vi "Dashboard Main.vi"() -> ()   [LabVIEW 2016]
uses:
  <vilib>/Rock Robotics/WPI/Camera/WPI_CameraSettings Read MJPG.ctl
  <vilib>/Rock Robotics/WPI/Camera/WPI_CameraImageSize.ctl
  HUD Time Slider.ctl
  <vilib>/Rock Robotics/WPI/DriverStation/WPI_DriverStationRobotMode2.ctl
  <vilib>/Rock Robotics/WPI/DriverStation/WPI_DriverStationAllianceInfo.ctl
  <vilib>/Rock Robotics/Network Tables/NT Read Numeric Array.vi
  <vilib>/Rock Robotics/Network Tables/NT Read Boolean.vi
  <vilib>/Rock Robotics/Network Tables/NT Write Numeric Array.vi
  <vilib>/event_ctls.llb/eventvkey.ctl
  <vilib>/Rock Robotics/WPI/Dashboard/WPI_DashboardLogging Global.vi
  <vilib>/Utility/miscctls.llb/LVRowAndColumnTypeDef.ctl
panel:
  out "CV LOCK":string
  out "Driver Control":bool
  out "Slide":T1 scale=0.0..100.0
  out "Robot Mode String":string
  out "Little Camera Image":T2(plugin-control)
  in  "TCP":refnum<k5>
  out "Robot IP":string
  out "Image Message":string="Timeout in Camera Communications"
  in  "Dashboard Tab":T3(tab)
  out "TALON ERR":bool
  out "VC ON":bool
  out "TEMP":dbl[unit](knob) scale=0.0..100.0
  out "AMPS":dbl(knob) caption="Gauge" scale=0.0..100.0
  out "Hopper Flaps":bool
  out "Hopper Down":bool
  out "Hopper Up":bool
  out "Intake Lock":bool
  out "Intake Active":bool
  out "Flaps":bool
  out "Gear Present":bool
  out "DeltaUS":dbl(knob) scale=-10.0..10.0
  out "ALIGN":bool caption="Boolean"
  out "Climb Motor Indicator":u32(colorbox)
  out "Intake Motor Indicator":u32(colorbox)
  out "Rear Right Indicator":u32(colorbox)
  out "Rear Left Indicator":u32(colorbox)
  out "Front Left Indicator":u32(colorbox)
  out "Front Right Indicator":u32(colorbox)
  out "BatPercentString":string
  out "BatteryPercent":u8(slide) scale=0.0..100.0
  out "BallSideActive":bool
  out "Mode":T4(ring)=enum."Auto Disabled"
  out "Gear is Front":bool
  out "Gear Auto Align":bool
  out "Auto Time Remaining":string
  out "INAV OK 2":bool
  out "CV OK":bool
  out "Auto Good":bool
  out "Robot Status":string
  out "Valid Autonomous Routines":i32(listbox)
  in  "AUTO SELECTION":i8(knob) scale=0.0..5.0
  out "Alliance Color":bool
  out "NT Connection":bool
  in  "Gear Side Camera Settings":T5={"fps"=30, "compression"=30, "Image Size"=enum."320x240", "Config Shown"=FALSE}
  in  "Ball Side Camera Settings":T5={"fps"=30, "compression"=30, "Image Size"=enum."320x240", "Config Shown"=FALSE}
  out "Ball Side Camera Info":cluster{bool, "Bandwidth (Mbps)":dbl, "FPS":dbl}
  out "Gear Side Camera Info":cluster{bool, "Bandwidth (Mbps)":dbl, "FPS":dbl}
  out "Big Camera Image":T2(plugin-control)
  # "HOPPER"
  # "A"
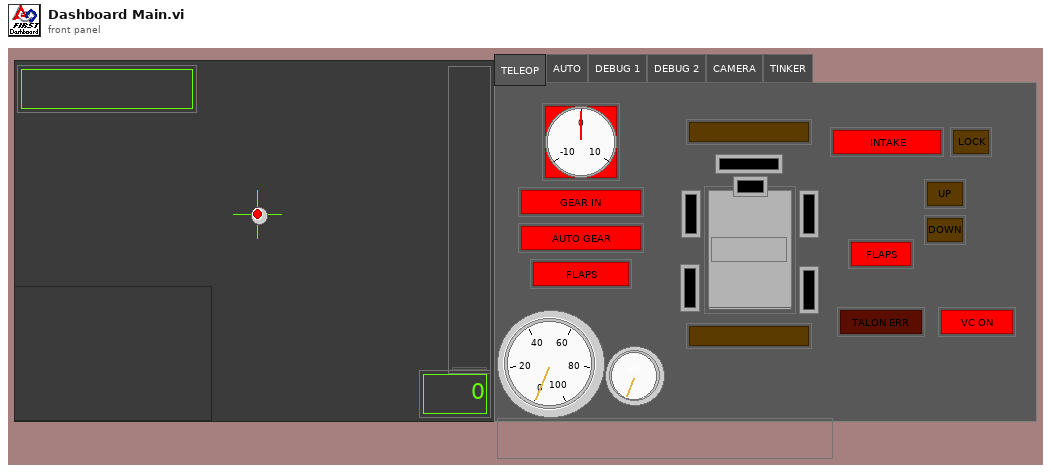
[diagram p1: front panel]
types:
  T1 = typedef "HUD Time Slider.ctl" = u8
  T2 = typedef "IMAQ Image.ctl" = refnum<image>
  T3 = enum32{"TELEOP", "AUTO", "DEBUG 1", "DEBUG 2", "CAMERA", "TINKER"}
  T4 = enum8{"Tele-Op Disabled", "Tele-Op Enabled", "Auto Disabled", "Auto Enabled", "Test Disabled", "Test Enabled", "Disconnected", "No Code", "E-Stop"}
  T5 = typedef "WPI_CameraSettings Read MJPG.ctl" = cluster{"fps":i32, "compression":i32, "Image Size":T6, "Config Shown":bool}
  T6 = typedef "WPI_CameraImageSize.ctl" = enum16{"640x480", "320x240", "160x120", "Custom"}
  T7 = typedef "Image Type" = u32
  T8 = cluster{"IDs":cluster{"RPC field ID":u16, "Unique ID":u16}, "String":string}
  T9 = enum32{"Drive", "Camera", "Basic", "Custom", "Test", "Commands", "Checklist", "Variables"}
  T10 = cluster{"Operation":enum16{"Update", "Clear"}, "Color Box":u32}[]
  T11 = typedef "eventvkey.ctl" = enum16{"ASCII", "Enter", "Return", "Shift", "Ctrl", "Alt", "Cmd", "Opt", "Caps", "NumLock", "Clear", "Break", "Up", "Down", "Left", "Right", "Insert", "Delete", "Home", "End", "PageUp", "PageDown", "Escape", "Help", "Pause", "ScrollLock", "F1", "F2", "F3", "F4", "F5", "F6", "F7", "F8", "F9", "F10", "F11", "F12", "F13", "F14", "F15", "F16", "F17", "F18", "F19", "F20", "F21", "F22", "F23", "F24", "Play", "VolumeUp", "VolumeDown", "Mute", "Two Byte Char"}
  T12 = cluster{"Image Size":bool, "Image Type":bool, "Pixel Value":bool, "ROI Information":bool, "Zoom Factor":bool}
  T13 = typedef "WPI_DriverStationRobotMode2.ctl" = enum16{"Autonomous Disabled", "Autonomous Enabled", "Teleop Disabled", "Teleop Enabled", "Disconnected", "Finish", "Test Disabled", "Test Enabled", "Emergency Stopped"}
  T14 = typedef "WPI_DriverStationAllianceInfo.ctl" = enum16{"Red", "Blue", "Invalid"}
  T15 = cluster{"Operation":enum16{"Update", "Clear"}, "Color Box":u32}
  T16 = typedef "LVRowAndColumnTypeDef.ctl" = cluster{"Row":i32, "Column":i32}
  T17 = cluster{"Test Progress":u8, "Test Progress Text":string}
  T18 = typedef "WPI_DriverStationPositionInfo.ctl" = enum16{"1", "2", "3"}
  T19 = cluster{"Error Strings":string, "Disable Counts":cluster{u16, u16}, "Rail Faults":cluster{u16, u16, u16}, "Robot IP":string, "DB Mode":u8, "Event Info":cluster{"Name":string, "Type":u8, "Number":u16, "Replay":u8}}
  T20 = cluster{"Storage":cluster{"Disk Free":u64, "RAM Block":u32, "RAM free":u32}, "CPU Utilization":cluster{"CPU % ISR":sgl, "CPU % Time Crit":sgl, "CPU % Timed Str":sgl, "CPU % High":sgl, "CPU % Above":sgl, "CPU % Normal":sgl, "CPU % Low":sgl}, "CAN":cluster{"% Bus Utilization":sgl, "Bus Off Cnt":u32, "TX_FIFO Full Cnt":u32, "Receive Error Cnt":u8, "Transmit Error Cnt":u8}, "HID":cluster{"HID Outputs":u32, "Rumble Low":u16, "Rumble High":u16}[]}
  T21 = cluster{"Status bits":cluster{"Test Mode":bool, "Autonomous":bool, "Enabled":bool, "Code Start":bool, "Brownout":bool, "Reserved 2":bool, "Reserved 3":bool, "E-Stop":bool}, "Code Trace":cluster{"Disabled":bool, "TeleOp":bool, "Auto":bool, "Test":bool}, "Controller Type":enum16{"unknown", "cRIO", "roboRio"}, "Code?":enum16{"unknown", "noCode", "code"}, "Battery V":dbl}
  T22 = cluster{"Control Bits":cluster{"TestMode":bool, "Autonomous":bool, "Enabled":bool, "FMS Present":bool, bool, bool, bool, "E-Stop":bool}, "Team Station ":u8, "Countdown":sgl, "Joystick Values":cluster{"Axes":dbl[], "Buttons":bool[], "POVs":i16[]}[]}
  T23 = cluster{"Axes":dbl[], "Buttons":bool[], "POVs":i16[]}[]
  T24 = cluster{"Axes":dbl[], "Buttons":bool[], "POVs":i16[]}
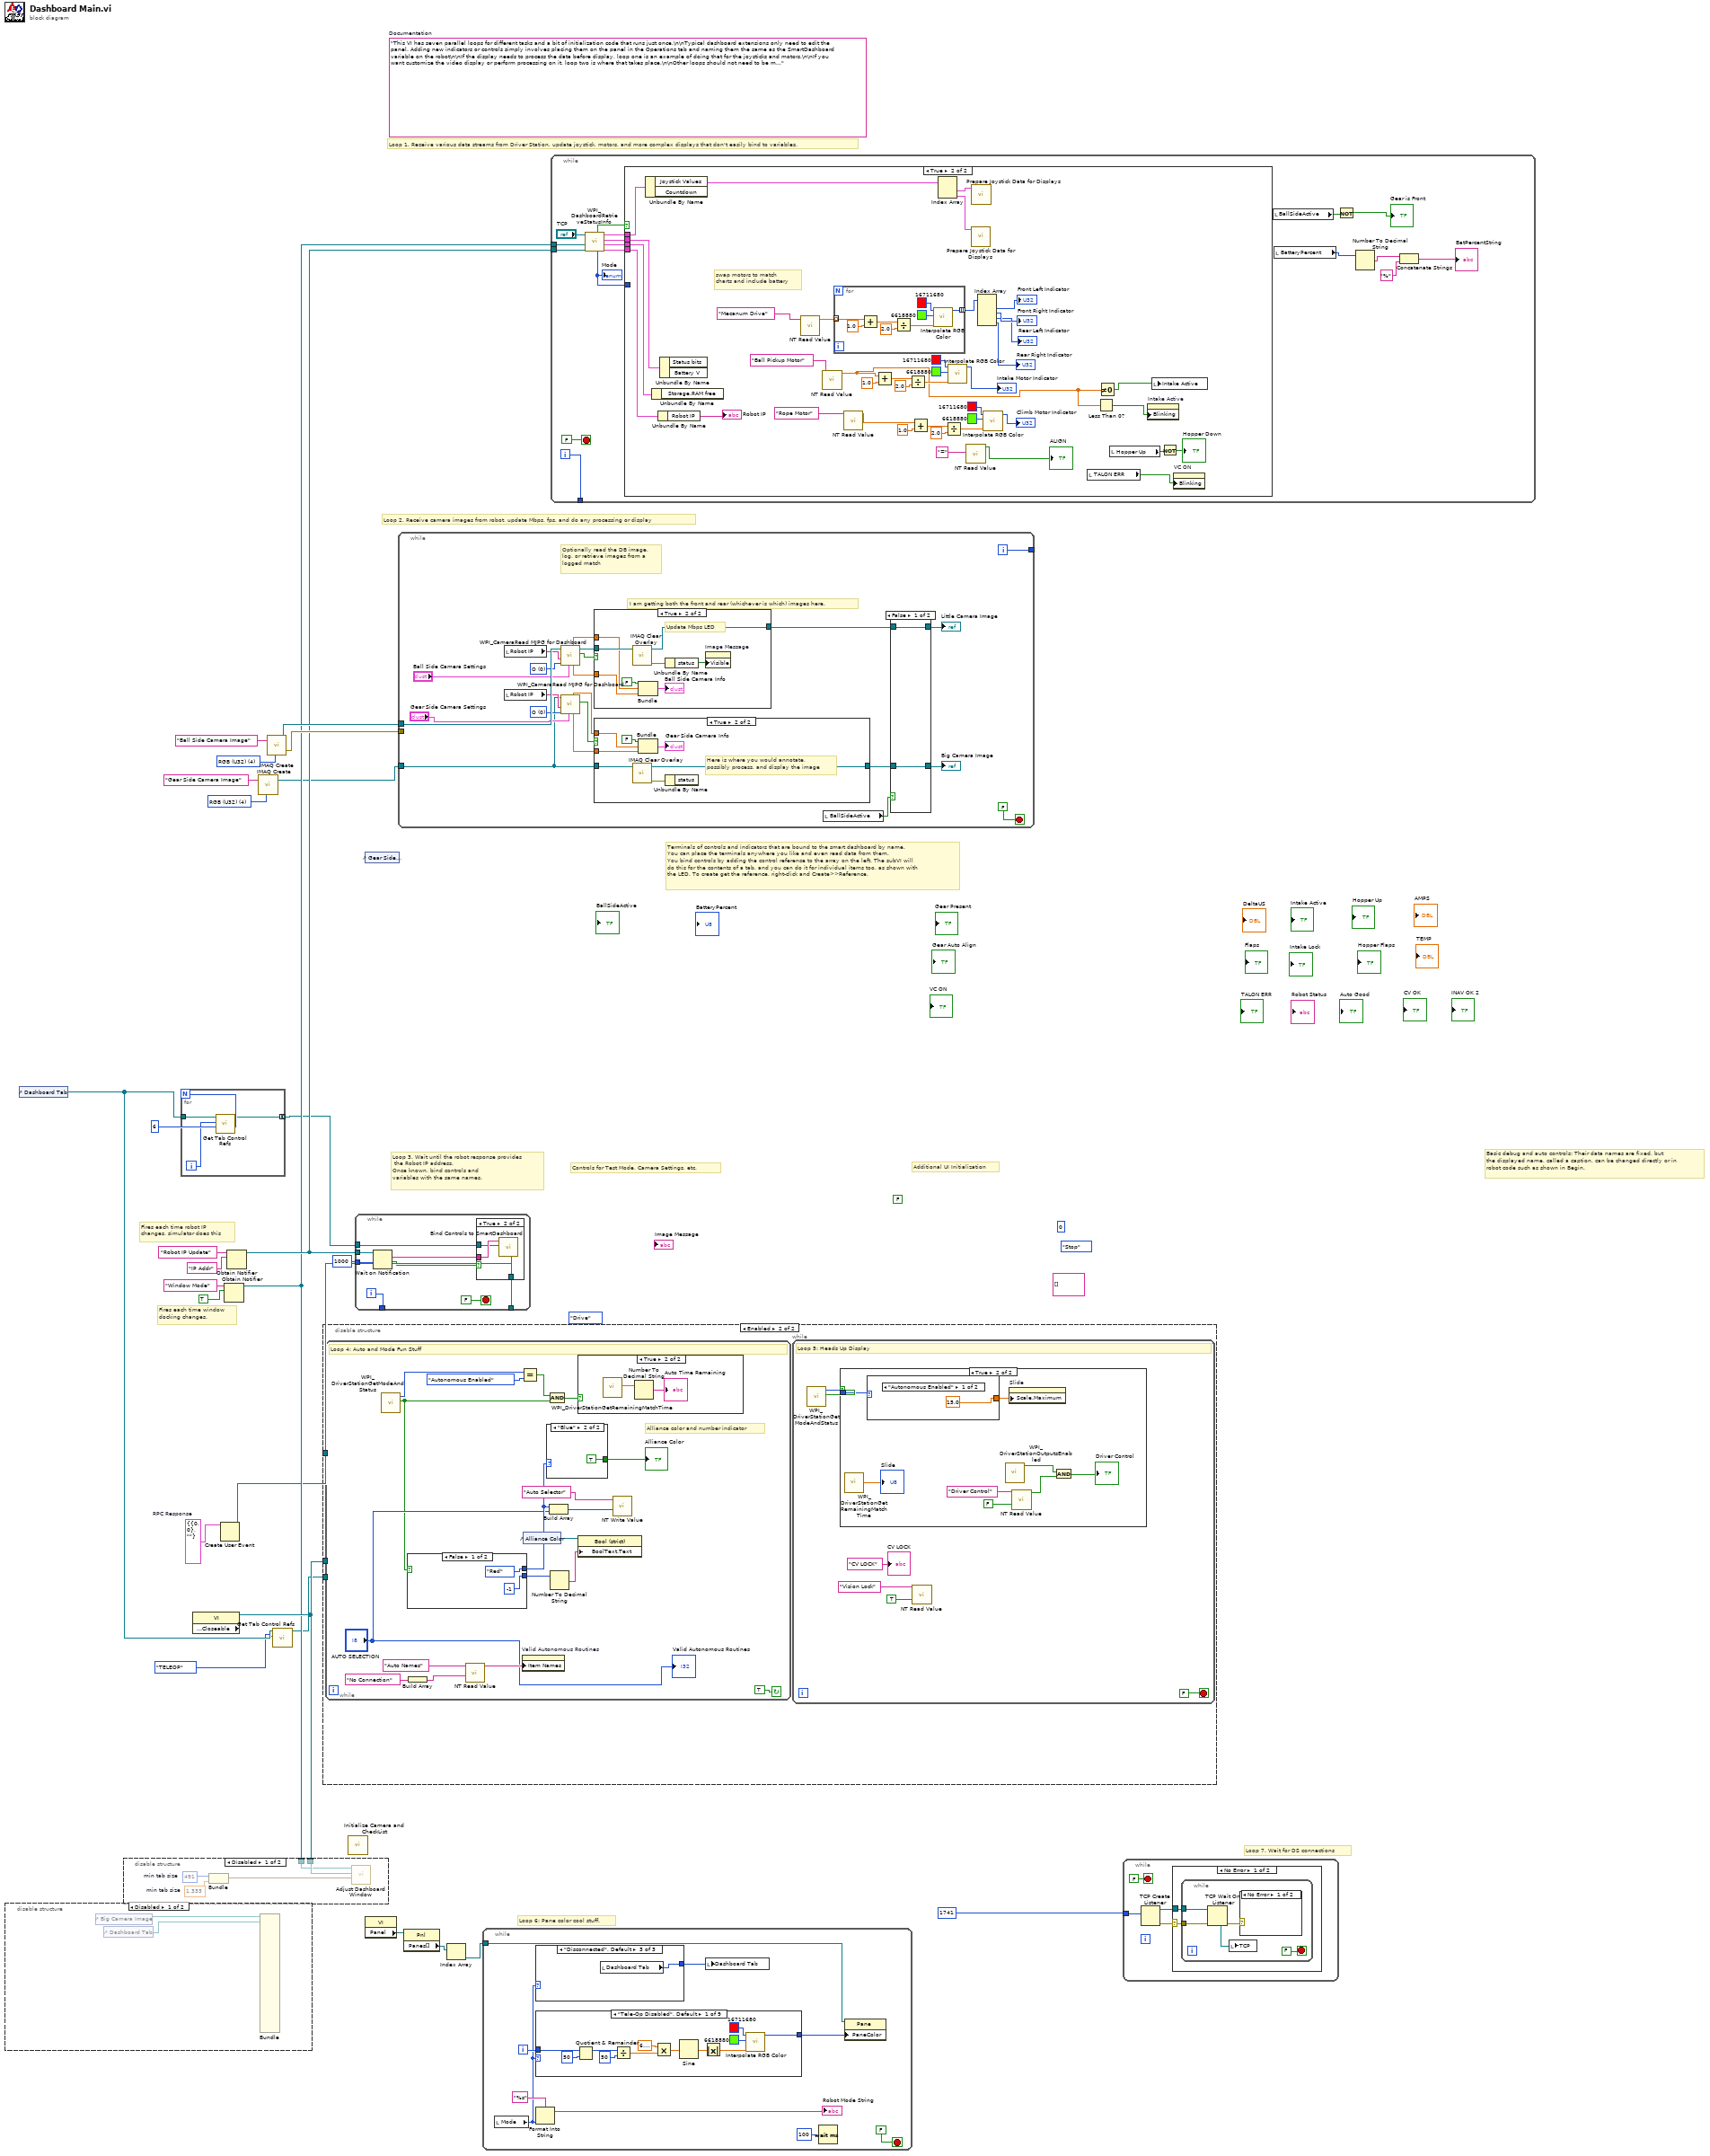
[diagram p0: block diagram]
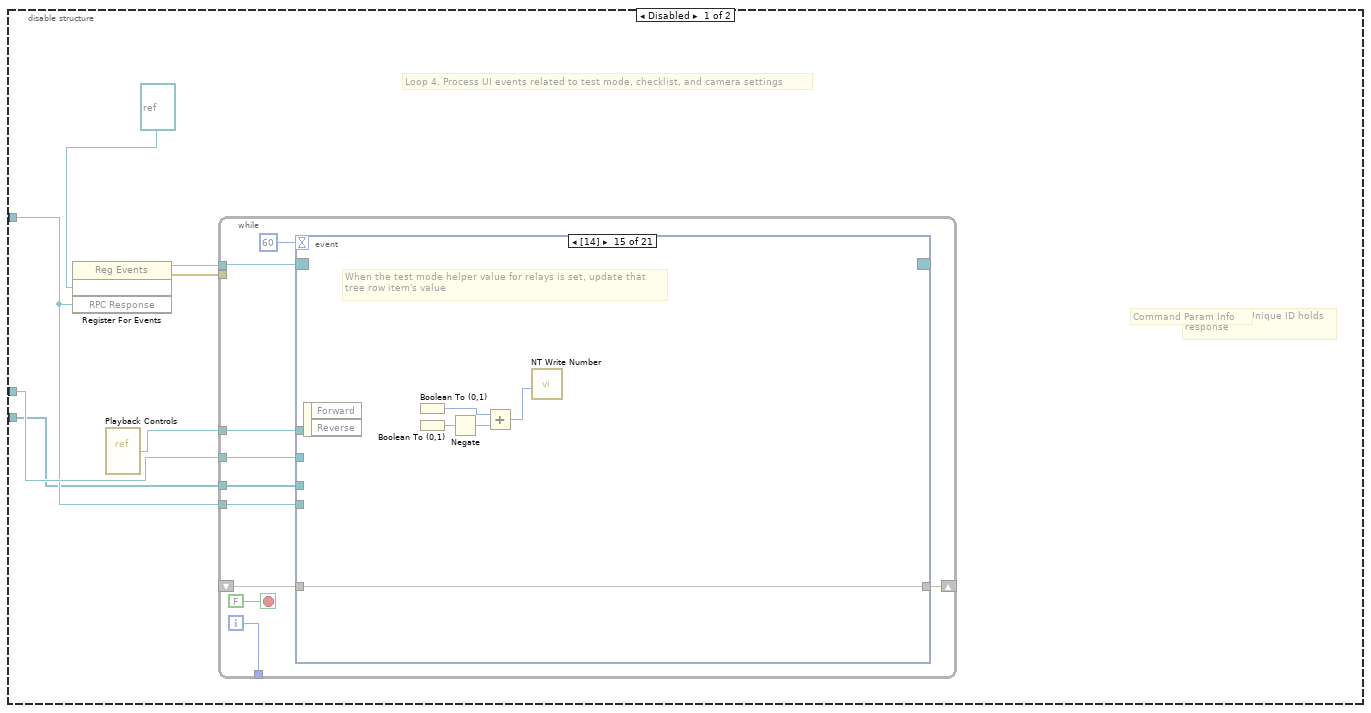
[diagram p4: hidden frame]
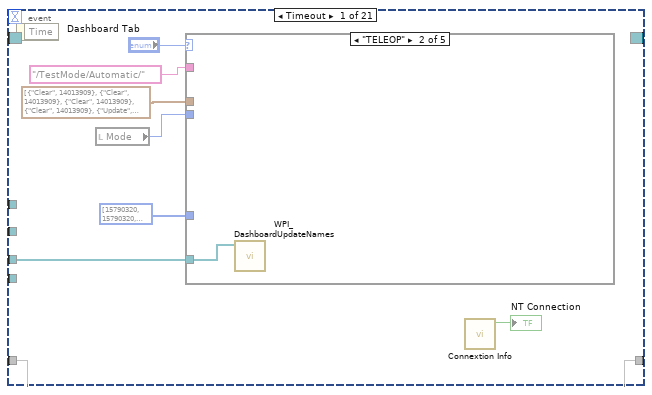
[diagram p5: hidden frame]
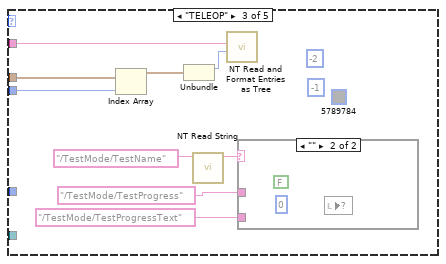
[diagram p7: hidden frame]
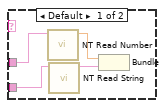
[diagram p8: hidden frame]
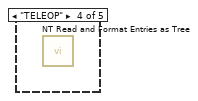
[diagram p9: hidden frame]
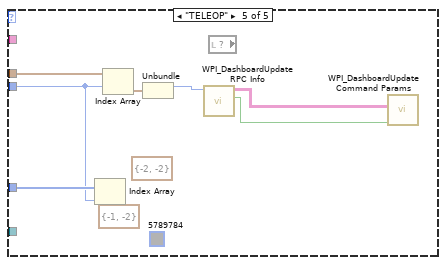
[diagram p10: hidden frame]
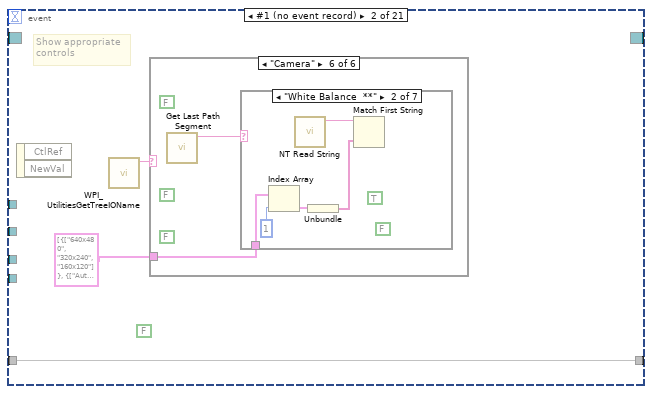
[diagram p11: hidden frame]
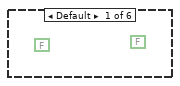
[diagram p12: hidden frame]
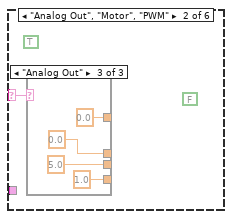
[diagram p13: hidden frame]
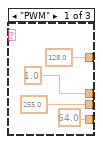
[diagram p14: hidden frame]
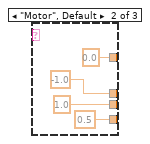
[diagram p15: hidden frame]
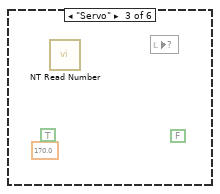
[diagram p16: hidden frame]
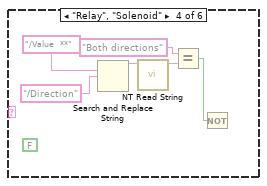
[diagram p17: hidden frame]
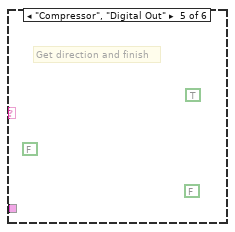
[diagram p18: hidden frame]
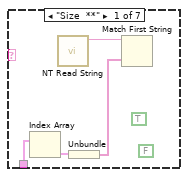
[diagram p19: hidden frame]
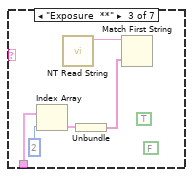
[diagram p20: hidden frame]
diagram:
  w8 = T7 4 items=["Grayscale (U8)", "Grayscale (I16)", "Grayscale (SGL)", "Complex (CSG)", "RGB (U32)", "HSL (U32)", "RGB (U64)"] ("Image Type")
  (unwired) u16 0 ("milliseconds to wait")
  (unwired) string[][] [] ("Command Params")
  w10 = T8 {"IDs"={"RPC field ID"=0, "Unique ID"=0}, "String"=""}  # RPC Response
  (unwired) T9."Drive" ("Dashboard Tab")
  (unwired) enum32{"Stop", "Record", "Playback"}."Stop" ("Rec Mode")
  (unwired) FALSE ("Visible")
  (unwired) "This VI has seven parallel loops for different tasks and a bit of initialization code that runs just once.\n\nTypical dashboard extensions only need to edit the panel. Adding new indicators or controls simply involves placing them on the panel in the Operations tab and naming them the same as the SmartDashboard variable on the robot\n\nIf the display needs to process the data before display, loop one is an example of doing that for the joysticks and motors.\n\nIf you want customize the video display or perform processing on it, loop two is where that takes place.\n\nOther loops should not need to be modified. They are pretty standard, and document the task they perform."  # Documentation
  w26 = T7 4 items=["Grayscale (U8)", "Grayscale (I16)", "Grayscale (SGL)", "Complex (CSG)", "RGB (U32)", "HSL (U32)", "RGB (U64)"] ("Image Type")
  # "Loop 7. Wait for DS connections"
  # "Basic debug and auto controls: Their data names are fixed, but\nthe displayed name, called a caption, can be changed directly or in\nrobot code such as shown in Begin."
  # "Controls for Test Mode, Camera Settings, etc."
  # "Additional UI Initialization"
  # "Loop 6: Pane color cool stuff."
  # "Fires each time robot IP\nchanges, simulator does this"
  # "Fires each time window\ndocking changes."
  # "Terminals of controls and indicators that are bound to the smart dashboard by name.\nYou can place the terminals anywhere you like and even read data from them.\nYou bind controls by adding the control reference to the array on the left. The subVI will\ndo this for the contents of a tab, and you can do it for individual items too, as shown with\nthe LED. To create get the reference, right-click and Create>>Reference."
  # "Loop 3. Wait until the robot response provides\n the Robot IP address.\nOnce known, bind controls and\nvariables with the same names."
  # "Loop 1. Receive various data streams from Driver Station, update joystick, motors, and more complex displays that don't easily bind to variables."
  # "Loop 2. Receive camera images from robot, update Mbps, fps, and do any processing or display"
  n1 = disable-structure shown="Disabled" {
    frame Disabled {
      n2 = control-ref of="Big Camera Image"() -> (w29:refnum<vi>)
      n3 = control-ref of="Dashboard Tab"() -> (w28:refnum<vi>)
      n4 = Bundle("Big Camera Image"=w29, "Dashboard Tab"=w28) -> (w27)  [unwired: 22 in, 1 out]
    }
    frame Enabled {
    }
  }
  n5 = control-ref of="Dashboard Tab"() -> (w2:refnum<vi>)
  n6 = for {
    N: 6 -> [_]
    tunnel: [w31] -> w3 mode=concatenating
    tunnel: w2 -> [w30]
    i -> [w32]
    n7 = call <vilib>:"Get Tab Control Refs.vi"("Page Index"=w32, "TabControl in"=w30) -> ("ControlsOnPage"=w31:refnum<vi>[])  [unwired: 9 in]
  }
  n8 = property class="VI" props=["Front Panel.Closeable"]() -> (reference out=w14:refnum<vi>)  [unwired: 2 in, 2 out]
  n9 = Create User Event(user event datatype=w10) -> (user event=w9:refnum<user-event>)  [unwired: 1 in, 1 out]
  n10 = Obtain Notifier(name (unnamed)="Window Mode", notification data type=TRUE) -> (notifier out=w12:refnum<notifier>)  [unwired: 2 in, 2 out]
  n11 = disable-structure shown="Disabled" {
    disable-tunnel: w14 -> [w37 _]
    disable-tunnel: w12 -> [w33 _]
    frame Disabled {
      w36 = 491  # min tab size
      w35 = 1.333  # min tab size
      n12 = Bundle("min tab size"=w36, "min tab size"=w35) -> (w34:cluster{"min tab size":i32, "min tab size":dbl})  [unwired: 1 in]
      n13 = call "Adjust Dashboard Window.vi"("Size Constraints"=w34, "VI"=w37, "WIn Mode"=w33) -> ()  [unwired: 9 in]
    }
    frame Enabled {
    }
  }
  n14 = Obtain Notifier(name (unnamed)="Robot IP Update", notification data type="IP Addr" ("name (unnamed)")) -> (notifier out=w13:refnum<notifier>)  [unwired: 2 in, 2 out]
  n15 = call "IMAQ Create"("Image Name"="Gear Side Camera Image", "Image Type"=w8) -> ("New Image"=w6:T2)  [unwired: 2 in, 2 out]
  n16 = call "IMAQ Create"("Image Name"="Ball Side Camera Image", "Image Type"=w26) -> ("New Image"=w24:T2, "error out"=w23:errorcluster)  [unwired: 2 in, 1 out]
  n17 = call <vilib>:"Get Tab Control Refs.vi"("Page Index"=T3."TELEOP" ("Dashboard Tab"), "TabControl in"=w2) -> ("ControlsOnPage"=w4:refnum<vi>[])  [unwired: 9 in]
  n18 = disable-structure shown="Enabled" {
    disable-tunnel: w14 -> [w40 _]
    disable-tunnel: w9 -> [w39 _]
    disable-tunnel: w4 -> [w38 _]
    frame Disabled {
      # "Command Param Info"
      # "Started one, Unique ID holds\nresponse"
      # "Loop 4. Process UI events related to test mode, checklist, and camera settings"
      n19 = register-events(refnum<vi> refnum, w39) -> (reference out=w43:refnum<event-registration>, error out=w42:errorcluster)  [unwired: 2 in]
      n20 = vi-ref "Playback Controls.vi"() -> (w44:refnum<vi>)
      n21 = while {
        tunnel: [w52] -> _
        tunnel: w44 -> [w51]
        tunnel: w43 -> [w50]
        tunnel: w42 -> [_]
        tunnel: w40 -> [w49]
        tunnel: w39 -> [w48]
        shift-right: [w47] -> _
        shift-left: _ -> [w46]
        tunnel: w38 -> [w45]
        i -> [w52]
        stop <- FALSE stop-if-true
        n22 = event shown="[14]" {
          selector: w50 -> [_ _ _ _ _ _ _ _ _ _ _ _ _ _ _ _ _ _ _ _ _]
          dyn-events: [_ _ _ _ _ _ _ _ _ _ _ _ _ _ _ _ w185 _ _ _ _] -> _
          timeout: u32 60 ("milliseconds to wait") -> [_ _ _ _ _ _ _ _ _ _ _ _ _ _ _ _ _ _ _ _ _]
          tunnel: w51 -> [_ _ _ _ _ _ _ _ _ _ _ _ _ _ _ _ w187 _ w205 _ _]
          tunnel: w49 -> [_ _ _ _ _ _ _ _ _ _ _ _ _ _ _ _ w183 _ _ _ _]
          tunnel: w48 -> [_ _ _ _ _ _ _ _ _ _ _ _ _ _ _ _ w179 _ _ _ _]
          tunnel: [w57 w85 w132 w136 w138 w141 w142 _ _ w153 w158 w166 w169 w170 w172 w177 w178 w200 w202 _ w211] -> w47
          tunnel: w46 -> [w57 w85 w132 w136 w138 w141 w142 _ _ w153 w158 w166 w169 w170 w172 w177 w178 w200 w202 _ w211]
          tunnel: w45 -> [w55 _ _ _ _ _ _ _ _ _ _ _ _ _ _ _ _ _ _ _ _]
          event Timeout {
            n23 = event-data() -> ()  [unwired: 1 in, 1 out]
            n24 = local read "Mode"() -> (w59:T4)
            n25 = case shown="\"Variables\"" "Dashboard Tab" {
              tunnel: "/TestMode/Automatic/" ("Name Pattern") -> [_ _ w72 _ _]
              tunnel: T10 [{"Operation"=enum."Clear", "Color Box"=14013909}, {"Operation"=enum."Clear", "Color Box"=14013909}, {"Operation"=enum."Clear", "Color Box"=14013909}, {"Operation"=enum."Clear", "Color Box"=14013909}, {"Operation"=enum."Update", "Color Box"=14013909}, {"Operation"=enum."Update", "Color Box"=16777215}, {"Operation"=enum."Clear", "Color Box"=14013909}, {"Operation"=enum."Clear", "Color Box"=14013909}, {"Operation"=enum."Clear", "Color Box"=14013909}] -> [_ _ w69 _ w82]
              tunnel: w59 -> [_ _ w68 _ w81]
              tunnel: u32[] [15790320, 15790320, 15790320, 15790320, 16777215, 16777215, 15790320, 15790320, 15790320] -> [_ _ _ _ w83]
              tunnel: w55 -> [_ w63 _ _ _]
              frame "TELEOP", Default {
              }
              frame "TELEOP" {
                n26 = call <vilib>:"WPI_DashboardUpdateNames.vi"("Controls on Tab"=w63) -> ()  [unwired: 11 in]
              }
              frame "TELEOP" {
                (unwired) u32 5789784 ("Color Box")
                (unwired) -1 ("Active Item:Row Number")
                (unwired) -2 ("Active Item:Row Number")
                n27 = Index Array(array=w69, index=w68) -> (element=w70:T15)
                n28 = Unbundle(w70) -> ("Operation"=w71:enum16{"Update", "Clear"})  [unwired: 1 out]
                n29 = call <vilib>:"NT Read String.vi"("Name"="/TestMode/TestName") -> ("String"=w66:string)  [unwired: 9 in, 1 out]
                n30 = call <vilib>:"NT Read and Format Entries as Tree.vi"("Operation"=w71, "Name Pattern"=w72) -> ()  [unwired: 8 in, 2 out]
                n31 = case shown="\"\"" w66 {
                  tunnel: "/TestMode/TestProgress" ("Name") -> [w74 _]
                  tunnel: "/TestMode/TestProgressText" ("Name") -> [w73 _]
                  frame Default {
                    n32 = call <vilib>:"NT Read Number.vi"("Name"=w74) -> ("Numeric"=w75:dbl)  [unwired: 9 in, 1 out]
                    n33 = call <vilib>:"NT Read String.vi"("Name"=w73) -> ("String"=w76:string)  [unwired: 9 in, 1 out]
                    n34 = Bundle("Numeric"=w75, "String"=w76) -> ()  [unwired: 1 in, 1 out]
                  }
                  frame "" {
                    (unwired) FALSE ("Visible")
                    (unwired) u16 0
                    n35 = local read item#-1() -> ()  [unwired: 1 in]
                  }
                }
              }
              frame "TELEOP" {
                n36 = call <vilib>:"NT Read and Format Entries as Tree.vi"() -> ()  [unwired: 10 in, 2 out]
              }
              frame "TELEOP" {
                (unwired) u32 5789784 ("Color Box")
                (unwired) T16 {"Row"=-1, "Column"=-2} ("Active Cell:Active Cell")
                (unwired) T16 {"Row"=-2, "Column"=-2} ("Active Cell:Active Cell")
                n37 = Index Array(array=w83, index=w81) -> ()  [unwired: 1 out]
                n38 = Index Array(array=w82, index=w81) -> (element=w80:T15)
                n39 = Unbundle(w80) -> ("Operation"=w79:enum16{"Update", "Clear"})  [unwired: 1 out]
                n40 = call <vilib>:"WPI_DashboardUpdate RPC Info.vi"("Operation"=w79) -> ("update"=w78:bool, "commands"=w77:string[][])  [unwired: 9 in]
                n41 = local read item#-1() -> ()  [unwired: 1 out]
                n42 = call <vilib>:"WPI_DashboardUpdate Command Params.vi"("Update"=w78, "Commands"=w77) -> ()  [unwired: 9 in, 1 out]
              }
            }
            n43 = call <vilib>:"Connextion Info.vi"() -> ("Connected"=→"NT Connection":bool)  [unwired: 10 in, 1 out]
          }
          event #1 (no event record) {
            (unwired) FALSE ("Visible")
            # "Show appropriate\ncontrols"
            n44 = event-data() -> ()  [unwired: 1 in, 2 out]
            n45 = call <vilib>:"WPI_UtilitiesGetTreeIOName.vi"() -> ("I/O Name"=w86:string)  [unwired: 11 in]
            n46 = case shown="\"Camera\"" w86 {
              selector: w86 -> [_ w87 _ _ _ _]
              tunnel: cluster{string[]}[] [{["640x480", "320x240", "160x120"]}, {["Auto", "Fixed indoor", "Fixed outdoor 1", "Fixed outdoor 2", "Fixed fluorescent 1", "Fixed fluorescent 2", "Hold current"]}, {["Auto", "Flicker-free 50 Hz", "Flicker-free 60 Hz", "Hold current"]}, {["None", "Prioritize frame rate", "Prioritize image quality"]}, {["Monochrome", "Color"]}] -> [_ _ _ _ _ w106]
              frame Default {
                (unwired) FALSE ("Visible")
                (unwired) FALSE ("Visible")
              }
              frame "Analog Out", "Motor", "PWM" {
                (unwired) FALSE ("Visible")
                (unwired) TRUE ("Visible")
                n47 = case shown="\"Analog Out\"" w87 {
                  tunnel: [1.0 ("Value") -1.0 ("Value") 0.0 ("Value")] -> _
                  tunnel: [255.0 ("Value") 1.0 ("Value") 5.0 ("Value")] -> _
                  tunnel: [128.0 ("Value") 0.0 ("Value") 0.0 ("Value")] -> _
                  tunnel: [64.0 ("Value") 0.5 ("Value") 1.0 ("Value")] -> _
                  frame "PWM" {
                  }
                  frame "Motor", Default {
                  }
                  frame "Analog Out" {
                  }
                }
              }
              frame "Servo" {
                (unwired) 170.0 ("Scale.Range:Maximum")
                (unwired) FALSE ("Visible")
                (unwired) TRUE ("Visible")
                n48 = call <vilib>:"NT Read Number.vi"() -> ()  [unwired: 10 in, 2 out]
                n49 = local read item#-1() -> ()  [unwired: 1 in]
              }
              frame "Relay", "Solenoid" {
                (unwired) FALSE ("Visible")
                n50 = Search and Replace String(search string="/Value  **", replace string="/Direction") -> (result string=w103:string)  [unwired: 6 in, 3 out]
                n51 = call <vilib>:"NT Read String.vi"("Name"=w103) -> ("String"=w101:string)  [unwired: 9 in, 1 out]
                n52 = Equal?(x="Both directions", y=w101) -> (x = y?=w100:bool)
                n53 = Not(x=w100) -> ()  [unwired: 1 out]
              }
              frame "Compressor", "Digital Out" {
                (unwired) FALSE ("Visible")
                (unwired) TRUE ("Visible")
                (unwired) FALSE ("Visible")
                # "Get direction and finish"
              }
              frame "Camera" {
                (unwired) FALSE ("Visible")
                (unwired) FALSE ("Visible")
                (unwired) FALSE ("Visible")
                n54 = call <vilib>:"Get Last Path Segment.vi"() -> ("String out"=w107:string)  [unwired: 11 in]
                n55 = case shown="\"White Balance  **\"" w107 {
                  tunnel: w106 -> [w110 w114 w119 w124 w129 _ _]
                  frame "Size  **" {
                    (unwired) FALSE ("Visible")
                    (unwired) TRUE ("Visible")
                    n56 = Index Array(array=w110) -> (element=w109:cluster{string[]})  [unwired: 1 in]
                    n57 = call <vilib>:"NT Read String.vi"() -> ("String"=w111:string)  [unwired: 10 in, 1 out]
                    n58 = Unbundle(w109) -> (w108:string[])
                    n59 = Match First String(2:w108, 3:w111) -> ()  [unwired: 2 out]
                  }
                  frame "White Balance  **" {
                    (unwired) FALSE ("Visible")
                    (unwired) TRUE ("Visible")
                    n60 = Index Array(array=w114, index=1) -> (element=w115:cluster{string[]})
                    n61 = call <vilib>:"NT Read String.vi"() -> ("String"=w116:string)  [unwired: 10 in, 1 out]
                    n62 = Unbundle(w115) -> (w112:string[])
                    n63 = Match First String(2:w112, 3:w116) -> ()  [unwired: 2 out]
                  }
                  frame "Exposure  **" {
                    (unwired) FALSE ("Visible")
                    (unwired) TRUE ("Visible")
                    n64 = Index Array(array=w119, index=2) -> (element=w120:cluster{string[]})
                    n65 = call <vilib>:"NT Read String.vi"() -> ("String"=w121:string)  [unwired: 10 in, 1 out]
                    n66 = Unbundle(w120) -> (w117:string[])
                    n67 = Match First String(2:w117, 3:w121) -> ()  [unwired: 2 out]
                  }
                  frame "Exposure Priority  **" {
                    (unwired) FALSE ("Visible")
                    (unwired) TRUE ("Visible")
                    n68 = Index Array(array=w124, index=3) -> (element=w125:cluster{string[]})
                    n69 = call <vilib>:"NT Read String.vi"() -> ("String"=w126:string)  [unwired: 10 in, 1 out]
                    n70 = Unbundle(w125) -> (w122:string[])
                    n71 = Match First String(2:w122, 3:w126) -> ()  [unwired: 2 out]
                  }
                  frame "Color Enable  **" {
                    (unwired) FALSE ("Visible")
                    (unwired) TRUE ("Visible")
                    n72 = Index Array(array=w129, index=4) -> (element=w130:cluster{string[]})
                    n73 = call <vilib>:"NT Read String.vi"() -> ("String"=w131:string)  [unwired: 10 in, 1 out]
                    n74 = Unbundle(w130) -> (w127:string[])
                    n75 = Match First String(2:w127, 3:w131) -> ()  [unwired: 2 out]
                  }
                  frame Default {
                    (unwired) FALSE ("Visible")
                    (unwired) FALSE ("Visible")
                  }
                  frame "Brightness  **", "Color Level  **", "Compression  **", "FPS  **", "Sharpness  **" {
                    (unwired) 100.0 ("Scale.Range:Maximum")
                    (unwired) FALSE ("Visible")
                    (unwired) TRUE ("Visible")
                    n76 = call <vilib>:"NT Read Number.vi"() -> ()  [unwired: 10 in, 2 out]
                    n77 = local read item#-1() -> ()  [unwired: 1 in]
                  }
                }
              }
            }
          }
          event #2 (no event record) {
            # "Populate the ring with the list of tests"
            n78 = event-data() -> ()  [unwired: 1 in, 1 out]
            n79 = call <vilib>:"NT Read String Array.vi"("Name"="/TestMode/TestList") -> ("String Array"=w135:string[])  [unwired: 9 in, 1 out]
            n80 = Build Array (concatenate)("Select the test to run...", w135) -> ()  [unwired: 1 out]
          }
          event #3 (no event record) {
            (unwired) FALSE ("Visible")
            (unwired) T17 {"Test Progress"=0, "Test Progress Text"=""} ("Progress")
            (unwired) TRUE ("Visible")
            # "Tell the robot the test name to run"
            n81 = event-data() -> ()  [unwired: 1 in, 1 out]
            n82 = local read item#-1() -> ()  [unwired: 1 in]
            n83 = Index Array() -> ()  [unwired: 2 in, 1 out]
            n84 = call <vilib>:"NT Write String.vi"("Name"="/TestMode/TestName") -> ()  [unwired: 10 in, 1 out]
          }
          event #4 (no event record) {
            # "Populate the combo box with the list of autonomous options"
            n85 = event-data() -> ()  [unwired: 1 in, 1 out]
            n86 = call <vilib>:"NT Read String Array.vi"("Name"="Auto List") -> ()  [unwired: 9 in, 2 out]
          }
          event #5 (no event record) {
            # "User modified the Auto Selection. Write to NT variable so robot knows."
            n87 = event-data() -> ()  [unwired: 1 in, 1 out]
            n88 = call <vilib>:"NT Write String.vi"("Name"="Auto Selector") -> ()  [unwired: 10 in, 1 out]
          }
          event #6 (no event record) {
            # "Get the params and show in table"
            n89 = event-data() -> ()  [unwired: 1 in, 1 out]
            n90 = call <vilib>:"WPI_DashboardUpdate Command Params.vi"() -> ()  [unwired: 11 in, 1 out]
          }
          event #7 (no event record) {
            # "Started one, Unique ID holds\nresponse"
            n91 = event-data() -> ()  [unwired: 1 in, 1 out]
            n92 = Index Array(index (col)=0) -> ()  [unwired: 2 in, 1 out]
            n93 = call <vilib>:"Invoke Commands.vi"() -> ("Params"=w146:u8, "Started"=w145:bool)  [unwired: 9 in, 1 out]
            n94 = Array Subset(length (row)=w146) -> ()  [unwired: 4 in, 1 out]
            n95 = Select(t="Executing" ("Cmd Status"), s=w145, f="" ("Cmd Status")) -> ()  [unwired: 1 out]
          }
          event #8 (no event record) {
            n96 = event-data() -> ()  [unwired: 1 in, 1 out]
            n97 = local read item#-1() -> ()  [unwired: 1 out]
            n98 = Index Array(index (col)=0) -> ()  [unwired: 2 in, 1 out]
            n99 = call <vilib>:"Invoke Commands.vi"() -> ("Params"=w151:u8, "Started"=w148:bool)  [unwired: 9 in, 1 out]
            n100 = Array Subset(length (row)=w151) -> ()  [unwired: 4 in, 1 out]
            n101 = Select(t="Executing" ("Cmd Status"), s=w148, f="" ("Cmd Status")) -> ()  [unwired: 1 out]
            n102 = local read item#-1() -> ()  [unwired: 1 in]
          }
          event #9 (no event record) {
            # "Shift clears all"
            # "Update symbols on the listbox"
            n103 = event-data() -> ("Row"=w155)  [unwired: 1 in, 1 out]
            n104 = case shown="True" {
              selector: _ -> [_ _]
              tunnel: w155 -> [_ _]
              tunnel: 1 -> [w156 _]
              frame False {
                n105 = Replace Array Subset(new element=w156) -> ()  [unwired: 2 in, 1 out]
              }
              frame True {
                (unwired) 0 ("Top Row")
                n106 = Initialize Array(0) -> ()  [unwired: 1 in, 1 out]
              }
            }
          }
          event #10 (no event record) {
            # "Update symbols on the listbox\nLeft and right keys check and uncheck"
            n107 = event-data() -> ()  [unwired: 1 in, 1 out]
            n108 = case shown="\"Left\", \"Right\"" {
              selector: _ -> [w164 _]
              tunnel: eventvkey."Left" ("VKey") -> [w162 _]
              frame "Left", "Right" {
                n109 = Equal?(x=w162, y=w164) -> (x = y?=w163:bool)
                n110 = Select(t=0, s=w163, f=1) -> (s? t:f=w165:i32)
                n111 = Replace Array Subset(new element=w165) -> ()  [unwired: 2 in, 1 out]
              }
              frame Default {
              }
            }
          }
          event #11 (no event record) {
            # "When the test mode otor enable helper is set, update that\ntree row item's value"
            n112 = event-data() -> ()  [unwired: 1 in, 1 out]
            n113 = Unbundle() -> ()  [unwired: 1 in, 2 out]
            n114 = Select(f=0.0) -> (s? t:f=w167:dbl)  [unwired: 2 in]
            n115 = call <vilib>:"NT Write Number.vi"("Numeric"=w167) -> ()  [unwired: 10 in, 1 out]
          }
          event #12 (no event record) {
            # "When the test mode slider helper is set, update that\ntree row item's value"
            n116 = event-data() -> ()  [unwired: 1 in, 1 out]
            n117 = call <vilib>:"NT Write Number.vi"() -> ()  [unwired: 11 in, 1 out]
          }
          event #13 (no event record) {
            # "When the test mode on/off helper value is set, update that\ntree row item's value"
            n118 = event-data() -> ()  [unwired: 1 in, 1 out]
            n119 = Boolean To (0,1)() -> (0, 1=w171:i16)  [unwired: 1 in]
            n120 = call <vilib>:"NT Write Number.vi"("Numeric"=w171) -> ()  [unwired: 10 in, 1 out]
          }
          event #14 (no event record) {
            # "When the test mode helper value for relays is set, update that\ntree row item's value"
            n121 = event-data() -> ()  [unwired: 1 in, 2 out]
            n122 = Boolean To (0,1)() -> (0, 1=w174:i16)  [unwired: 1 in]
            n123 = Boolean To (0,1)() -> (0, 1=w176:i16)  [unwired: 1 in]
            n124 = Negate(x=w176) -> (-x=w175:i16)
            n125 = Add(x=w174, y=w175) -> (x+y=w173:i16)
            n126 = call <vilib>:"NT Write Number.vi"("Numeric"=w173) -> ()  [unwired: 10 in, 1 out]
          }
          event #15 (no event record) {
            # "When a test mode helper value is selected from the ring,\nset the tree item's variable to the string value"
            n127 = event-data() -> ()  [unwired: 1 in, 1 out]
            n128 = Index Array() -> ()  [unwired: 2 in, 1 out]
            n129 = call <vilib>:"NT Write String.vi"() -> ()  [unwired: 11 in, 1 out]
          }
          event #16 (no event record) {
            # "Update globals for recording mode and path to read log from.\nClear when logging and let NetworkTables set path for vision to\nuse."
            n130 = event-data() -> ("NewVal"=w188)  [unwired: 1 in]
            n131 = global write "WPI_DashboardLogging Global.vi" "Logging Filename"(path "") -> ()
            n132 = global write "WPI_DashboardLogging Global.vi" "Recording"(w188) -> ()
            n133 = case shown="\"Playback\"" w188 {
              tunnel: w187 -> [_ w190 w199]
              tunnel: [_ _ w198] -> w185
              tunnel: [_ _ w197] -> _
              tunnel: w183 -> [_ _ w195]
              tunnel: cluster{i32, i32} {-250, 170} -> [_ _ w194]
              tunnel: [_ _ T12 {"Image Size"=TRUE, "Image Type"=TRUE, "Pixel Value"=TRUE, "ROI Information"=TRUE, "Zoom Factor"=FALSE} ("Image Information Shown:All Elements")] -> w181
              tunnel: [_ _ TRUE ("Zoom Factor")] -> w180
              tunnel: w179 -> [_ _ w191]
              frame Default {
              }
              frame "Stop", "Record" {
                # "Place Window too"
                n134 = invoke class="VI" method="FP.Close"(reference=w190) -> (reference out=w189:refnum<vi>)  [unwired: 2 in, 2 out]
                n135 = invoke class="VI" method="Abort VI"(reference=w189) -> ()  [unwired: 2 in, 3 out]
              }
              frame "Playback" {
                n136 = call "Open Playback Panel.vi"("Offset"=w194, "DB VI Ref"=w195, "Playback in"=w199) -> ("Playback out"=w196:refnum<vi>)  [unwired: 8 in]
                n137 = register-events(w196, w191) -> (reference out=w198:refnum<event-registration>, error out=w197:errorcluster)  [unwired: 2 in]
              }
            }
            n138 = property on="Big Camera Image" class="ImageControl"("Image Information Shown"=w181, "Image Information Visible"=w180) -> ()  [unwired: 2 in, 2 out]
            n139 = call <vilib>:"WPI_DashboardNT Log FieldName Cache.vi"("Operation"=enum16{"Lookup/Add", "Index", "Clear"}."Clear") -> ()  [unwired: 8 in, 3 out]
          }
          event Panel Close {
            w201 = enum32{"Stop", "Record", "Playback"}."Stop" ("Rec Mode")
            # "Playback window has been closed, abort"
            n140 = event-data() -> ()  [unwired: 1 in, 4 out]
            n141 = global write "WPI_DashboardLogging Global.vi" "Recording"(w201) -> ()
            n142 = local write item#-1(w201) -> ()
          }
          event Panel Close {
            # "Abort playback window and ourself"
            n143 = event-data() -> ()  [unwired: 1 in, 4 out]
            n144 = invoke class="VI" method="FP.Close"(reference=w205) -> (reference out=w204:refnum<vi>)  [unwired: 2 in, 2 out]
            n145 = invoke class="VI" method="Abort VI"(reference=w204) -> (error out=w203:errorcluster)  [unwired: 2 in, 2 out]
            n146 = invoke class="VI" method="Abort VI"(error in=w203) -> ()  [unwired: 2 in, 3 out]
          }
          event User Event {
            (unwired) "" ("Cmd Status")
            n147 = event-data() -> ("IDs"=w209:cluster{"RPC field ID":u16, "Unique ID":u16}, "String"=w208:string)  [unwired: 1 in]
            n148 = Bundle("IDs"=w209, "String"=w208) -> (w207:T8)  [unwired: 1 in]
            n149 = call <vilib>:"Retrieve RPC Response.vi"("RPC Response"=w207) -> ("Output"=w206:string[][])  [unwired: 10 in]
            n150 = Build Array (concatenate)(w206) -> ()  [unwired: 1 in, 1 out]
            n151 = local read item#-1() -> ()  [unwired: 1 in]
            n152 = local read item#-1() -> ()  [unwired: 1 in]
          }
          event #20 (no event record) {
            n153 = event-data() -> ()  [unwired: 1 in, 2 out]
            n154 = Unbundle() -> ()  [unwired: 1 in, 5 out]
            n155 = Not() -> (.not. x?=w210:bool)  [unwired: 1 in]
            n156 = call <vilib>:"NT Update Persistence.vi"("Persistence"=w210) -> ()  [unwired: 10 in, 1 out]
          }
        }
      }
    }
    frame Enabled {
      n157 = while {
        stop <- TRUE continue-if-true
        # "Alliance color and number indicator"
        # "Loop 4: Auto and Mode Fun Stuff"
        n158 = call <vilib>:"WPI_DriverStationGetModeAndStatus.vi"() -> ("FMS Attached"=w229:bool, "Robot Mode"=w232:T13)  [unwired: 10 in]
        n159 = case shown="False" w229 {
          tunnel: [-1 w251] -> w244
          tunnel: [WPI_DriverStationAllianceInfo."Red" ("Alliance") w250] -> w240
          frame False {
          }
          frame True {
            n160 = call <vilib>:"WPI_DriverStationGet Alliance Info.vi"() -> ("Position"=w251:T18, "Alliance"=w250:T14)  [unwired: 10 in]
          }
        }
        n161 = Build Array("No Connection") -> (w235:string[])
        n162 = call-poly <vilib>:"NT Read Value.vi"("Default Value"=w235, "Name"="Auto Names") -> ("String Array"=w238:string[])  [unwired: 8 in, 1 out]
        n163 = Equal?(x=w232, y=WPI_DriverStationRobotMode2."Autonomous Enabled") -> (x = y?=w230:bool)
        n164 = property on="Valid Autonomous Routines" class="LstBox (strict)"("Item Names"=w238) -> ()  [unwired: 2 in, 2 out]
        n165 = control-ref of="Alliance Color"() -> (w245:refnum<vi>)
        n166 = case shown="\"Blue\"" w240 {
          tunnel: [FALSE TRUE] -> w242
          frame "Red", Default {
          }
          frame "Blue" {
          }
        }
        "Alliance Color" <- w242
        n167 = And(x=w230, y=w229) -> (x .and. y?=w228:bool)
        n168 = Build Array(w240, "AUTO SELECTION") -> (w239:u16[])
        n169 = Number To Decimal String(number=w244) -> (decimal integer string=w243:string)  [unwired: 1 in]
        n170 = case shown="True" w228 {
          frame False {
          }
          frame True {
            n171 = call <vilib>:"WPI_DriverStationGetRemainingMatchTime.vi"() -> ("Match Time(s)"=w247:sgl)  [unwired: 10 in, 1 out]
            n172 = Number To Decimal String(number=w247) -> (decimal integer string=→"Auto Time Remaining":string)  [unwired: 1 in]
          }
        }
        n173 = property class="Bool (strict)"(reference=w245, "BoolText.Text"=w243) -> ()  [unwired: 1 in, 2 out]
        n174 = call-poly <vilib>:"NT Write Value.vi"("Numeric Array"=w239, "Name"="Auto Selector") -> ()  [unwired: 9 in, 1 out]
        "Valid Autonomous Routines" <- "AUTO SELECTION"
      }
      n175 = while {
        stop <- FALSE stop-if-true
        # "Loop 5: Heads Up Display"
        n176 = call <vilib>:"WPI_DriverStationGetModeAndStatus.vi"() -> ("FMS Attached"=w216:bool, "Robot Mode"=w217:T13)  [unwired: 10 in]
        n177 = case shown="True" w216 {
          tunnel: w217 -> [_ w225]
          frame False {
          }
          frame True {
            n178 = call <vilib>:"WPI_DriverStationGetRemainingMatchTime.vi"() -> ("Match Time(s)"=→"Slide":sgl)  [unwired: 10 in, 1 out]
            n179 = case shown="\"Autonomous Enabled\"" w225 {
              tunnel: [15.0 135.0 ("Scale.Range:Maximum")] -> w224
              frame "Autonomous Enabled" {
              }
              frame "Teleop Enabled", Default {
              }
            }
            n180 = call <vilib>:"WPI_DriverStationOutputsEnabled.vi"() -> ("OutputsEnabled?"=w219:bool)  [unwired: 10 in, 1 out]
            n181 = property on="Slide" class="Slide (strict)"("Scale.Maximum"=w224) -> ()  [unwired: 2 in, 2 out]
            n182 = call-poly <vilib>:"NT Read Value.vi"("Default Value"=FALSE, "Name"="Driver Control") -> ("Boolean"=w221:bool)  [unwired: 8 in, 1 out]
            n183 = And(x=w219, y=w221) -> (x .and. y?=→"Driver Control":bool)
          }
        }
        n184 = call-poly <vilib>:"NT Read Value.vi"("Default Value"=TRUE, "Name"="Vision Lock") -> ()  [unwired: 8 in, 2 out]
        "CV LOCK" <- "CV LOCK" ("CV LOCK")
      }
    }
  }
  n185 = call "Initialize Camera and CheckList.vi"() -> ()  [unwired: 12 in]
  n186 = while {
    tunnel: w13 -> [w260]
    tunnel: [w258] -> _
    tunnel: u32 1000 ("milliseconds to wait") -> [w257]
    tunnel: w9 -> [w256]
    tunnel: w3 -> [w255]
    i -> [w258]
    stop <- FALSE stop-if-true
    n187 = Wait on Notification(notifier=w260, timeout in ms (-1)=w257) -> (notification=w259:string, timed out?=w254:bool)  [unwired: 2 in, 2 out]
    n188 = case shown="True" w254 {
      tunnel: w259 -> [_ w264]
      tunnel: w256 -> [_ w263]
      tunnel: w255 -> [_ w262]
      frame False {
      }
      frame True {
        n189 = call <vilib>:"Bind Controls to SmartDashboard.vi"("RPC ref"=w263, "Bound Control Refs"=w262, "Server IP Address"=w264) -> ()  [unwired: 9 in]
      }
    }
  }
  n190 = control-ref of="Gear Side Camera Settings"() -> ()  [unwired: 1 out]
  n191 = property class="VI"() -> ("Panel"=w17:refnum<vi>)  [unwired: 2 in, 2 out]
  n192 = while {
    tunnel: w24 -> [w284]
    tunnel: w23 -> [_]
    tunnel: [w285] -> _
    tunnel: w6 -> [w265]
    i -> [w285]
    stop <- FALSE stop-if-true
    w266 = u16 0 items=["O", "*", "Open Playback Panel"] ("Rec Mode")
    w267 = u16 0 items=["O", "*", "Open Playback Panel"] ("Rec Mode")
    # "I am getting both the front and rear (whichever is which) images here."
    # "Optionally read the DB image,\nlog, or retrieve images from a\nlogged match"
    n193 = local read "Robot IP"() -> (w280:string)
    n194 = local read "Robot IP"() -> (w273:string)
    n195 = call <vilib>:"WPI_CameraRead MJPG for Dashboard.vi"("Camera Settings"="Ball Side Camera Settings", "Rec Mode"=w267, "Robot IP"=w280, "Refnum in"=w284) -> ("Active"=w282:bool, "Refnum out"=w283:T2, "FPS"=w281:dbl, "Bandwidth (Mbps)"=w279:dbl)  [unwired: 4 in]
    n196 = call <vilib>:"WPI_CameraRead MJPG for Dashboard.vi"("Camera Settings"="Gear Side Camera Settings", "Rec Mode"=w266, "Robot IP"=w273, "Refnum in"=w265) -> ("Active"=w277:bool, "FPS"=w275:dbl, "Bandwidth (Mbps)"=w276:dbl)  [unwired: 4 in, 1 out]
    n197 = case shown="True" w282 {
      tunnel: w283 -> [w302 w311]
      tunnel: w279 -> [_ w309]
      tunnel: w281 -> [_ w310]
      tunnel: [w302 w307] -> w271
      frame False {
        w303 = u32 1985280 ("Color Box")
        # "Sleep for 500ms"
        n198 = Bundle("Color Box"=w303, "Color Box"=w303) -> (w304:cluster{"Color Box":u32, "Color Box":u32})  [unwired: 1 out]
        n199 = Wait Until Next ms Multiple(millisecond multiple=u32 500) -> ()  [unwired: 1 out]
        n200 = Build Array(w304) -> ()  [unwired: 1 out]
      }
      frame True {
        # "Update Mbps LED"
        n201 = call "IMAQ Clear Overlay"("Image"=w311) -> ("error out"=w312:errorcluster, "Image Out"=w307:T2)  [unwired: 2 in, 7 out]
        n202 = Bundle(FALSE, "Bandwidth (Mbps)"=w309, "FPS"=w310) -> (→"Ball Side Camera Info":cluster{bool, "Bandwidth (Mbps)":dbl, "FPS":dbl})  [unwired: 1 in]
        n203 = Unbundle By Name(w312) -> ("status"=w313:bool)
        n204 = property on="Image Message" class="Str"("Visible"=w313) -> ()  [unwired: 2 in, 2 out]
      }
    }
    n205 = case shown="True" w277 {
      tunnel: w265 -> [w291 w300]
      tunnel: w275 -> [_ w299]
      tunnel: [w291 w297] -> w270
      tunnel: w276 -> [_ w296]
      frame False {
        w292 = u32 1985280 ("Color Box")
        # "Sleep for 500ms"
        n206 = Bundle("Color Box"=w292, "Color Box"=w292) -> (w293:cluster{"Color Box":u32, "Color Box":u32})  [unwired: 1 out]
        n207 = Wait Until Next ms Multiple(millisecond multiple=u32 500) -> ()  [unwired: 1 out]
        n208 = Build Array(w293) -> ()  [unwired: 1 out]
      }
      frame True {
        # "Here is where you would annotate,\npossibly process, and display the image"
        n209 = call "IMAQ Clear Overlay"("Image"=w300) -> ("error out"=w301:errorcluster, "Image Out"=w297:T2)  [unwired: 2 in, 7 out]
        n210 = Bundle(FALSE, "Bandwidth (Mbps)"=w296, "FPS"=w299) -> (→"Gear Side Camera Info":cluster{bool, "Bandwidth (Mbps)":dbl, "FPS":dbl})  [unwired: 1 in]
        n211 = Unbundle By Name(w301) -> ()  [unwired: 1 out]
      }
    }
    n212 = local read "BallSideActive"() -> (w272:bool)
    n213 = case shown="False" w272 {
      tunnel: w271 -> [w288 w289]
      tunnel: w270 -> [w287 w290]
      tunnel: [w288 w290] -> w269
      tunnel: [w287 w289] -> w268
      frame False {
      }
      frame True {
      }
    }
    "Little Camera Image" <- w269
    "Big Camera Image" <- w268
  }
  n214 = property class="Pnl"(reference=w17) -> ("Panes[]"=w18:refnum<vi>[])  [unwired: 1 in, 2 out]
  n215 = Index Array(array=w18) -> (element=w16:refnum<vi>)  [unwired: 1 in]
  n216 = while {
    tunnel: w16 -> [w319]
    i -> [w321]
    stop <- FALSE stop-if-true
    n217 = local read "Mode"() -> (w315:T4)
    n218 = case shown="\"Disconnected\", Default" w315 {
      tunnel: [T3."TELEOP" ("Dashboard Tab") T3."AUTO" ("Dashboard Tab") w325] -> w314
      frame "Tele-Op Enabled" {
      }
      frame "Auto Enabled" {
      }
      frame "Disconnected", Default {
        n219 = local read "Dashboard Tab"() -> (w325:T3)
      }
    }
    n220 = case shown="\"Tele-Op Disabled\", Default" w315 {
      selector: w315 -> [_ _ _ _ w353 _ _ _ _]
      tunnel: w321 -> [w327 _ w350 _ _ _ w366 w378 _]
      tunnel: [w326 u32 6618880 ("Target Color") w339 u32 9567230 ("Target Color") w352 u32 16716509 ("Base Color") w365 w377 u32 16711680 ("Target Color")] -> w318
      frame "Tele-Op Disabled", Default {
        n221 = Quotient & Remainder(x=w327, y=u32 50 ("milliseconds to wait")) -> (x-y*floor(x/y)=w334:u32)  [unwired: 1 out]
        n222 = Divide(x=w334, y=u32 50 ("milliseconds to wait")) -> (x/y=w331:dbl)
        n223 = Multiply(x=6.283185307179586, y=w331) -> (x*y=w336:dbl)
        n224 = Sine(x=w336) -> (sin(x)=w335:dbl)
        n225 = Absolute Value(x=w335) -> (abs(x)=w328:dbl)
        n226 = call "Interpolate RGB Color.vi"("Proportion"=w328, "Target Color"=u32 6618880, "Base Color"=u32 16711680) -> ("Result Color"=w326:u32)  [unwired: 8 in]
      }
      frame "Tele-Op Enabled" {
      }
      frame "Auto Disabled" {
        n227 = Quotient & Remainder(x=w350, y=u32 50 ("milliseconds to wait")) -> (x-y*floor(x/y)=w346:u32)  [unwired: 1 out]
        n228 = Divide(x=w346, y=u32 50 ("milliseconds to wait")) -> (x/y=w343:dbl)
        n229 = Multiply(x=6.283185307179586, y=w343) -> (x*y=w348:dbl)
        n230 = Sine(x=w348) -> (sin(x)=w347:dbl)
        n231 = Absolute Value(x=w347) -> (abs(x)=w340:dbl)
        n232 = call "Interpolate RGB Color.vi"("Proportion"=w340, "Target Color"=u32 9567230, "Base Color"=u32 16711680) -> ("Result Color"=w339:u32)  [unwired: 8 in]
      }
      frame "Auto Enabled" {
      }
      frame "Test Disabled" {
        n233 = Quotient & Remainder(x=w353, y=u32 50 ("milliseconds to wait")) -> (x-y*floor(x/y)=w360:u32)  [unwired: 1 out]
        n234 = Divide(x=w360, y=u32 50 ("milliseconds to wait")) -> (x/y=w357:dbl)
        n235 = Multiply(x=6.283185307179586, y=w357) -> (x*y=w362:dbl)
        n236 = Sine(x=w362) -> (sin(x)=w361:dbl)
        n237 = Absolute Value(x=w361) -> (abs(x)=w354:dbl)
        n238 = call "Interpolate RGB Color.vi"("Proportion"=w354, "Target Color"=u32 16711680, "Base Color"=u32 16716509) -> ("Result Color"=w352:u32)  [unwired: 8 in]
      }
      frame "Test Enabled" {
      }
      frame "Disconnected" {
        n239 = Quotient & Remainder(x=w366, y=u32 50 ("milliseconds to wait")) -> (x-y*floor(x/y)=w373:u32)  [unwired: 1 out]
        n240 = Divide(x=w373, y=u32 50 ("milliseconds to wait")) -> (x/y=w370:dbl)
        n241 = Multiply(x=6.283185307179586, y=w370) -> (x*y=w375:dbl)
        n242 = Sine(x=w375) -> (sin(x)=w374:dbl)
        n243 = Absolute Value(x=w374) -> (abs(x)=w367:dbl)
        n244 = call "Interpolate RGB Color.vi"("Proportion"=w367, "Target Color"=u32 9868950, "Base Color"=u32 16711680) -> ("Result Color"=w365:u32)  [unwired: 8 in]
      }
      frame "No Code" {
        n245 = Quotient & Remainder(x=w378, y=u32 50 ("milliseconds to wait")) -> (x-y*floor(x/y)=w385:u32)  [unwired: 1 out]
        n246 = Divide(x=w385, y=u32 50 ("milliseconds to wait")) -> (x/y=w382:dbl)
        n247 = Multiply(x=6.283185307179586, y=w382) -> (x*y=w387:dbl)
        n248 = Sine(x=w387) -> (sin(x)=w386:dbl)
        n249 = Absolute Value(x=w386) -> (abs(x)=w379:dbl)
        n250 = call "Interpolate RGB Color.vi"("Proportion"=w379, "Target Color"=u32 0, "Base Color"=u32 16749312) -> ("Result Color"=w377:u32)  [unwired: 8 in]
      }
      frame "E-Stop" {
      }
    }
    n251 = Format Into String "Format Into String"(format string="%s", w315) -> (resulting string=→"Robot Mode String":string)  [unwired: 2 in, 1 out]
    n252 = local write "Dashboard Tab"(w314) -> ()
    n253 = Wait (ms)(milliseconds to wait=u32 100) -> ()  [unwired: 1 out]
    n254 = property class="Pane"(reference=w319, "PaneColor"=w318) -> ()  [unwired: 1 in, 2 out]
  }
  n255 = while {
    tunnel: [w405] -> _
    tunnel: w13 -> [w399]
    tunnel: w12 -> [w396]
    i -> [w405]
    stop <- FALSE stop-if-true
    n256 = call <vilib>:"WPI_DashboardRetrieveStatusInfo.vi"("Binding Refnum"=w399, "Window Mode Notifier"=w396, "TCP Cnx"="TCP") -> ("Power and Errors"=w400:T19, "Robot Metrics"=w403:T20, "Status Info"=w404:T21, "Control Info"=w401:T22, "Robot Mode"=w398:T4, "Process?"=w402:bool)  [unwired: 3 in]
    "Mode" <- w398
    n257 = case shown="True" w402 {
      tunnel: w404 -> [_ w447]
      tunnel: w403 -> [_ w446]
      tunnel: w401 -> [_ w445]
      tunnel: w400 -> [_ w444]
      tunnel: w398 -> [_ _]
      frame False {
        n258 = Wait (ms)(milliseconds to wait=u32 20) -> ()  [unwired: 1 out]
      }
      frame True {
        # "swap motors to match\ncharts and include battery"
        n259 = Unbundle By Name(w445) -> ("Joystick Values"=w443:T23)  [unwired: 1 out]
        n260 = Unbundle By Name(w446) -> ()  [unwired: 1 out]
        n261 = Unbundle By Name(w444) -> ("Robot IP"=→"Robot IP":string)
        n262 = Unbundle By Name(w447) -> ()  [unwired: 2 out]
        n263 = call-poly <vilib>:"NT Read Value.vi"("Name"="Mecanum Drive") -> ("Numeric Array"=w438:dbl[])  [unwired: 9 in, 1 out]
        n264 = call-poly <vilib>:"NT Read Value.vi"("Name"="Ball Pickup Motor") -> ("Numeric"=w413:dbl)  [unwired: 9 in, 1 out]
        n265 = for {
          tunnel: w438 -> [w455] mode=indexing
          tunnel: [w448] -> w436 mode=indexing
          n266 = Add(x=w455, y=1.0) -> (x+y=w453:dbl)
          n267 = Divide(x=w453, y=2.0) -> (x/y=w451:dbl)
          n268 = call "Interpolate RGB Color.vi"("Proportion"=w451, "Target Color"=u32 6618880, "Base Color"=u32 16711680) -> ("Result Color"=w448:u32)  [unwired: 8 in]
        }
        n269 = call-poly <vilib>:"NT Read Value.vi"("Name"="Rope Motor") -> ("Numeric"=w419:dbl)  [unwired: 9 in, 1 out]
        n270 = Add(x=w413, y=1.0) -> (x+y=w430:dbl)
        n271 = Divide(x=w430, y=2.0) -> (x/y=w428:dbl)
        n272 = Add(x=w419, y=1.0) -> (x+y=w424:dbl)
        n273 = Index Array(array=w443) -> (element #1=w442:T24, element #2=w441:T24)  [unwired: 2 in]
        n274 = Divide(x=w424, y=2.0) -> (x/y=w422:dbl)
        n275 = call "Interpolate RGB Color.vi"("Proportion"=w428, "Target Color"=u32 6618880, "Base Color"=u32 16711680) -> ("Result Color"=→"Intake Motor Indicator":u32)  [unwired: 8 in]
        n276 = call-poly <vilib>:"NT Read Value.vi"("Name"="=") -> ("Boolean"=→"ALIGN":bool)  [unwired: 9 in, 1 out]
        n277 = call "Prepare Joystick Data for Displays.vi"("Joystick Values"=w441) -> ()  [unwired: 8 in, 3 out]
        n278 = call "Prepare Joystick Data for Displays.vi"("Joystick Values"=w442) -> ()  [unwired: 8 in, 3 out]
        n279 = Index Array(array=w436) -> (element #1=→"Front Left Indicator":u32, element #2=→"Front Right Indicator":u32, element #3=→"Rear Left Indicator":u32, element #4=→"Rear Right Indicator":u32)  [unwired: 4 in]
        n280 = call "Interpolate RGB Color.vi"("Proportion"=w422, "Target Color"=u32 6618880, "Base Color"=u32 16711680) -> ("Result Color"=→"Climb Motor Indicator":u32)  [unwired: 8 in]
        n281 = local read "TALON ERR"() -> (w409:bool)
        n282 = Less Than 0?(x=w413) -> (x < 0?=w412:bool)
        n283 = Not Equal To 0?(x=w413) -> (x != 0?=w414:bool)
        n284 = local read "Hopper Up"() -> (w410:bool)
        n285 = property on="Intake Active" class="Bool (strict)"("Blinking"=w412) -> ()  [unwired: 2 in, 2 out]
        n286 = local write "Intake Active"(w414) -> ()
        n287 = Not(x=w410) -> (.not. x?=→"Hopper Down":bool)
        n288 = property on="VC ON" class="Bool (strict)"("Blinking"=w409) -> ()  [unwired: 2 in, 2 out]
      }
    }
    n289 = local read "BallSideActive"() -> (w395:bool)
    n290 = local read "BatteryPercent"() -> (w393:u8)
    n291 = Not(x=w395) -> (.not. x?=→"Gear is Front":bool)
    n292 = Number To Decimal String(number=w393) -> (decimal integer string=w392:string)  [unwired: 1 in]
    n293 = Concatenate Strings(w392, "%" ("string")) -> (→"BatPercentString":string)
  }
  n294 = while {
    tunnel: u16 1741 ("timeout ms (25000)") -> [w457]
    stop <- FALSE stop-if-true
    n295 = TCP Create Listener(10:w457) -> (0:w456:errorcluster, 3:w458:refnum<k5>)  [unwired: 4 in, 1 out]
    n296 = case shown="No Error" w456 {
      selector: w456 -> [w460 _]
      tunnel: w458 -> [w461 _]
      frame No Error {
        n297 = while {
          tunnel: w461 -> [w464]
          tunnel: w460 -> [w463]
          stop <- FALSE stop-if-true
          n298 = TCP Wait On Listener(8:w463, 11:w464) -> (0:w465:errorcluster, 4:w466:refnum<k5>)  [unwired: 2 in, 3 out]
          n299 = local write "TCP"(w466) -> ()
          n300 = case shown="No Error" w465 {
            frame No Error {
            }
            frame Error {
              n301 = Wait (ms)(milliseconds to wait=u32 1000) -> ()  [unwired: 1 out]
            }
          }
        }
      }
      frame Error {
        n302 = Wait (ms)(milliseconds to wait=u32 1000) -> ()  [unwired: 1 out]
      }
    }
  }
